vi "Set Wheel Separation.vi"(6 "subpanel to main command event":T1, 8 "error in (no error)":errorcluster, 10 "wheel separation":dbl, 11 "steering frame ref in":refnum<data-value>) -> (0 "error out":errorcluster, 3 "steering frame ref out":refnum<data-value>)   [LabVIEW 2017, in "NI_Robotics_Configure Steering Frame.lvlib" / "Differential Frame Subpanel.lvlib"]
uses:
  <vilib>/robotics/Dialog/Configure Steering Frame/Differential Frame Subpanel/Differential Frame Subpanel.lvlib
  <vilib>/robotics/Steering/Differential Steering Frame/NI_Robotics_Differential Steering Frame.lvclass
  c:/Program Files (x86)/National Instruments/LabVIEW 2017/vi.lib/robotics/Steering/Steering Frame/NI_Robotics_Steering Frame.lvclass
  <vilib>/robotics/Dialog/Configure Steering Frame/Subpanel to Main Command Event.ctl
  <vilib>/robotics/Dialog/Configure Steering Frame/Subpanel to Main Command.ctl
  <vilib>/robotics/Steering/Steering Frame/NI_Robotics_Steering Frame.lvclass/NI_Robotics_Steering Frame.ctl
  <vilib>/robotics/Steering/Wheel/NI_Robotics_Wheel.lvclass/NI_Robotics_Wheel.ctl
  <vilib>/robotics/Steering/Differential Steering Frame/NI_Robotics_Differential Steering Frame.lvclass/NI_Robotics_Differential Steering Frame.ctl
  <vilib>/robotics/Steering/Differential Steering Frame/Wheel Separation to Frame Positions.vi
  <vilib>/robotics/Steering/Steering Frame/Reposition Wheels.vi
  <vilib>/robotics/Dialog/Configure Steering Frame/Generate Subpanel to Main Event.vi
  <vilib>/robotics/Steering/Wheel/Update Steering to Wheel Frame Transform.vi
  <vilib>/Analysis/coordinate.llb/Wrap Angle.vi
  <vilib>/Analysis/coordinate.llb/Wrap Angle (scalar).vi
  <vilib>/robotics/Dialog/Configure Steering Frame/NI_Robotics_Configure Steering Frame.lvlib
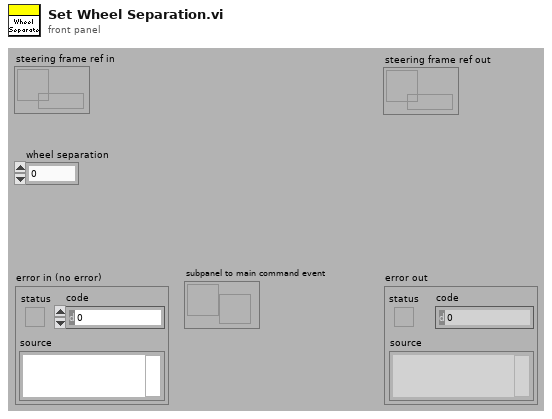
[diagram p1: front panel]
types:
  T1 = typedef "NI_Robotics_Configure Steering Frame.lvlib/Subpanel to Main Command Event.ctl" = refnum<user-event>
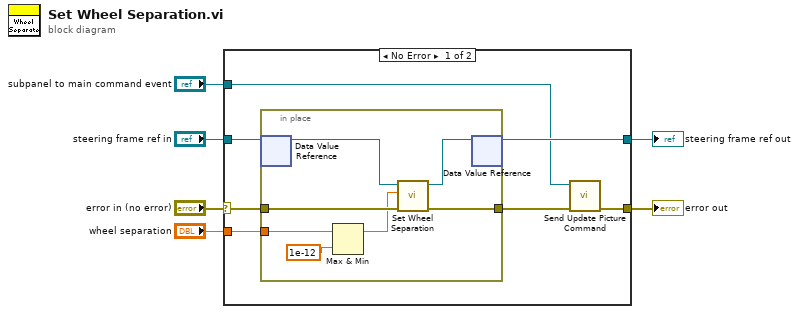
[diagram p0: block diagram]
diagram:
  n1 = case shown="No Error" "error in (no error)" {
    selector: "error in (no error)" -> [w11 w21]
    tunnel: "steering frame ref in" -> [w13 w22]
    tunnel: [w12 w22] -> w4
    tunnel: [w7 w21] -> w3
    tunnel: "wheel separation" -> [w10 _]
    tunnel: "subpanel to main command event" -> [w9 _]
    frame No Error {
      n2 = in-place {
        in-place-border: w11 -> [w18]
        in-place-border: [w17] -> w8
        in-place-border: w10 -> [w15]
        n3 = in-place-dvr #1(w13) -> (w20:refnum<class "NI_Robotics_Differential Steering Frame.lvclass">)  [unwired: 1 out]
        n4 = Max & Min(x=w15, y=1e-12) -> (max(x,y)=w14:dbl)  [unwired: 1 out]
        n5 = call <vilib>:"Set Wheel Separation.vi"("error in (no error)"=w18, "wheel separation"=w14, "differential steering frame in"=w20) -> ("error out"=w17:errorcluster, "differential steering frame out"=w19:refnum<class "NI_Robotics_Differential Steering Frame.lvclass">)  [unwired: 7 in]
        n6 = in-place-dvr #1(w19) -> (w12:refnum<data-value>)  [unwired: 1 out]
      }
      n7 = call <vilib>:"Send Update Picture Command.vi"("error in (no error)"=w8, "subpanel to main command event"=w9) -> ("error out"=w7:errorcluster)  [unwired: 9 in]
    }
    frame Error {
    }
  }
  "steering frame ref out" <- w4
  "error out" <- w3
